vi "ShooterSpeedToConfigEnum.vi"(1 "ShooterSpeed":dbl) -> (0 "ConfigEnum":T1)   [LabVIEW 2016]
uses:
  TypeDefs/ShooterSpeed_Type.ctl
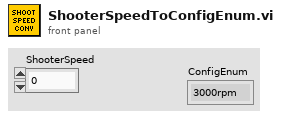
[diagram p1: front panel]
types:
  T1 = typedef "ShooterSpeed_Type.ctl" = enum16{"3000rpm", "3500rpm", "4000rpm", "4500rpm", "5000rpm", "FullPower"}
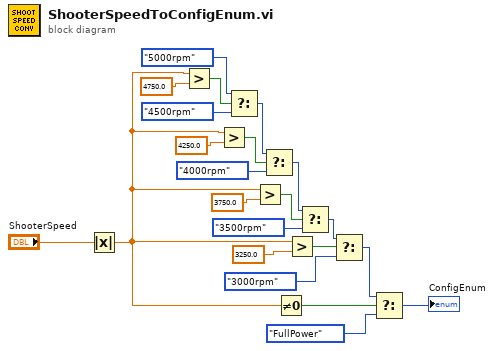
[diagram p0: block diagram]
diagram:
  n1 = Absolute Value(x="ShooterSpeed") -> (abs(x)=w5:dbl)
  n2 = Greater?(x=w5, y=4750.0) -> (0:w9:bool)
  n3 = Greater?(x=w5, y=4250.0) -> (0:w13:bool)
  n4 = Select(t=ShooterSpeed_Type."5000rpm", s=w9, f=ShooterSpeed_Type."4500rpm" ("ConfigEnum 2")) -> (s? t:f=w7:T1)
  n5 = Greater?(x=w5, y=3750.0) -> (0:w17:bool)
  n6 = Select(t=w7, s=w13, f=ShooterSpeed_Type."4000rpm" ("ConfigEnum 2")) -> (s? t:f=w11:T1)
  n7 = Not Equal To 0?(x=w5) -> (x != 0?=w3:bool)
  n8 = Greater?(x=w5, y=3250.0) -> (0:w20:bool)
  n9 = Select(t=w11, s=w17, f=ShooterSpeed_Type."3500rpm" ("ConfigEnum 2")) -> (s? t:f=w16:T1)
  n10 = Select(t=w16, s=w20, f=ShooterSpeed_Type."3000rpm" ("ConfigEnum 2")) -> (s? t:f=w4:T1)
  n11 = Select(t=w4, s=w3, f=ShooterSpeed_Type."FullPower") -> (s? t:f=→"ConfigEnum":T1)
